vi "Configure Session.vi"(8 "error in":errorcluster, 11 "Plugin in":refnum<class "RIO Streamer.lvclass">) -> (0 "error out":errorcluster, 3 "Plugin out":refnum<class "RIO Streamer.lvclass">)   [LabVIEW 2024, in "RIO Streamer.lvlib" / "RIO Streamer.lvclass"]
uses:
  RIO Streamer.lvclass
  C:/Program Files/National Instruments/LabVIEW 2024/vi.lib/FlexLogger/SDK/PluginSDK.lvlibp/PEFClasses/SDK/Plugin/Plugin.lvclass
  RIO Streamer.lvclass/RIO Streamer.ctl
  <vilib>/FlexLogger/SDK/PluginSDK.lvlibp/PEFClasses/SDK/Channel/ParameterAccess/Read DBL.vi
  <vilib>/FlexLogger/SDK/PluginSDK.lvlibp/PEFClasses/SDK/Plugin/ParameterAccess/Read String.vi
  <vilib>/FlexLogger/SDK/PluginSDK.lvlibp/PEFClasses/SDK/Plugin/ParameterAccess/Read DBL.vi
  <vilib>/FlexLogger/SDK/PluginSDK.lvlibp/PEFClasses/SDK/Plugin/Plugin.lvclass
  <vilib>/FlexLogger/SDK/PluginSDK.lvlibp/PEFClasses/SDK/Channel/Channel.lvclass
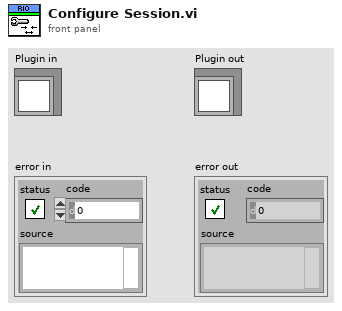
[diagram p1: front panel]
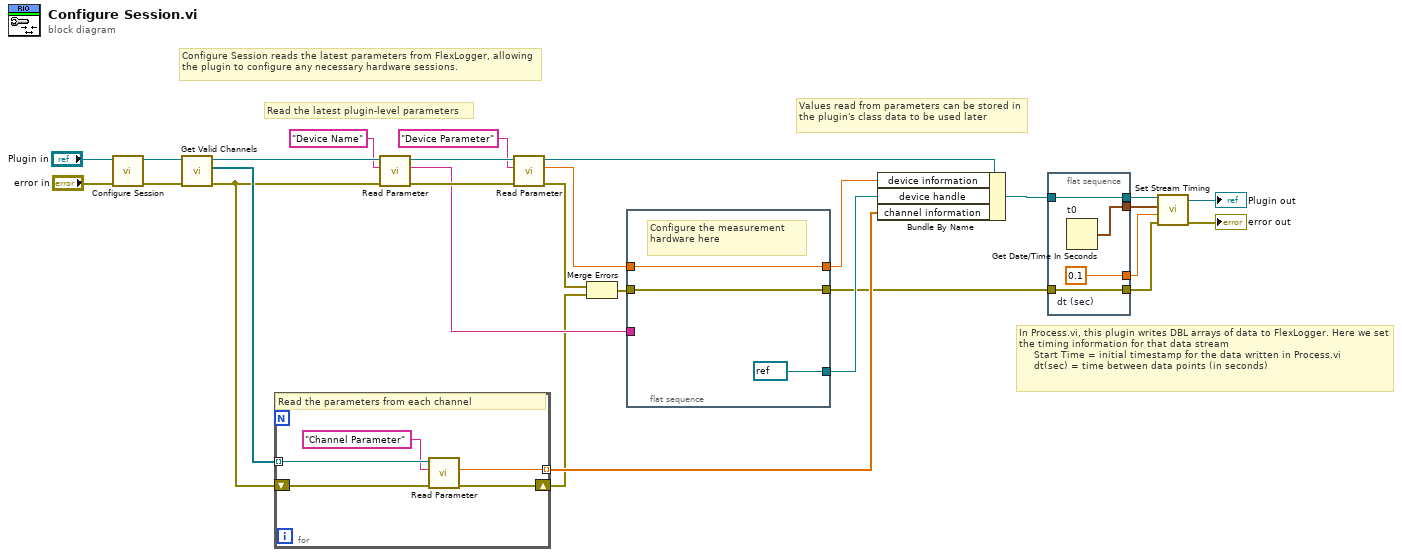
[diagram p0: block diagram]
diagram:
  # "Read the latest plugin-level parameters"
  # "Configure Session reads the latest parameters from FlexLogger, allowing the plugin to configure any necessary hardware sessions."
  # "Values read from parameters can be stored in the plugin's class data to be used later"
  # "In Process.vi, this plugin writes DBL arrays of data to FlexLogger. Here we set the timing information for that data stream\n     Start Time = initial timestamp for the data written in Process.vi\n     dt(sec) = time between data points (in seconds)"
  n1 = call-parent "Configure Session.vi"("error in (no error)"="error in", "Processing Element in"="Plugin in") -> ("error out"=w18:errorcluster, "Processing Element out"=w19:refnum<class "RIO Streamer.lvclass">)  [unwired: 8 in]
  n2 = call <vilib>:"Get Valid Channels.vi"("error in (no error)"=w18, "Plugin in"=w19) -> ("error out"=w4:errorcluster, "Channels"=w26:refnum<class "Channel.lvclass">[], "Plugin out"=w25:refnum<class "RIO Streamer.lvclass">)  [unwired: 7 in]
  n3 = for {
    tunnel: w26 -> [w33] mode=indexing
    tunnel: [w31] -> w17 mode=indexing
    shift-right: [w30] -> w7
    shift-left: w4 -> [w29]
    # "Read the parameters from each channel"
    n4 = call-poly <vilib>:"Read Parameter.vi"("error in (no error)"=w29, "Name"="Channel Parameter", "Channel in"=w33) -> ("error out"=w30:errorcluster, "Value"=w31:dbl)  [unwired: 5 in, 2 out]
  }
  n5 = call-poly <vilib>:"Read Parameter.vi"("error in (no error)"=w4, "Name"="Device Name", "Plugin in"=w25) -> ("error out"=w23:errorcluster, "Value"=w14:string, "Plugin out"=w24:refnum<class "RIO Streamer.lvclass">)  [unwired: 5 in, 1 out]
  n6 = call-poly <vilib>:"Read Parameter.vi"("error in (no error)"=w23, "Name"="Device Parameter", "Plugin in"=w24) -> ("error out"=w6:errorcluster, "Value"=w16:dbl, "Plugin out"=w21:refnum<class "RIO Streamer.lvclass">)  [unwired: 5 in, 1 out]
  n7 = Merge Errors(w6, w7) -> (w5:errorcluster)
  n8 = flat-sequence {
    tunnel: [w36] -> w12
    tunnel: w5 -> [w36]
    tunnel: w16 -> [w34]
    tunnel: [refnum<k15> refnum ("device handle")] -> w15
    tunnel: w14 -> [_]
    tunnel: [w34] -> w3
    frame #0 {
      # "Configure the measurement hardware here"
    }
  }
  n9 = Bundle By Name(cluster=w21, "device information"=w3, "device handle"=w15, "channel information"=w17) -> (w13:refnum<class "RIO Streamer.lvclass">)
  n10 = flat-sequence {
    tunnel: [w40] -> w10
    tunnel: [w39] -> w8
    tunnel: w12 -> [w38]
    tunnel: [w38] -> w9
    tunnel: w13 -> [w37]
    tunnel: [w37] -> w11
    frame #0 {
      w39 = 0.1  # dt (sec)
      n11 = Get Date/Time In Seconds "t0"() -> (seconds since 1Jan1904=w40:timestamp)
    }
  }
  n12 = call-dynamic "Set Stream Timing.vi"("error in (no error)"=w9, "dt(sec)"=w8, "Start Time"=w10, "Plugin in"=w11) -> ("error out"=→"error out":errorcluster, "Plugin out"=→"Plugin out":refnum<class "RIO Streamer.lvclass">)  [unwired: 6 in]
